vi "Download File to Stream.vi"(6 "timeout (ms)":i32=30000, 8 "error in":errorcluster, 10 "remote path":string, 11 "session in":refnum<class "Session.lvclass">) -> (0 "error out":errorcluster, 2 "channel":T1, 3 "session out":refnum<class "Session.lvclass">)   [LabVIEW 2020, in "NI_SFTP.lvlib"]
doc: "Downloads a remote file, returning the contents as a High-Speed Stream of byte arrays."
uses:
  <vilib>/net/SFTP/NI_SFTP.lvlib
  <vilib>/net/SFTP/Session/Session.lvclass
  <extravilib>/ChannelInstances/High Speed Stream-a[.](u8)/)Channel.ctl
  <vilib>/ChannelSupport/Channel Abort Instructions.ctl
  <extravilib>/ChannelInstances/High Speed Stream-a[.](u8)/)Channel.vi
  <vilib>/net/SFTP/API/Support/Download/Stream/Stream Download Controller.lvclass
  <vilib>/Utility/Deadline/NI_Deadline.lvlib
  <extravilib>/ChannelInstances/High Speed Stream-a[.](u8).lvlib
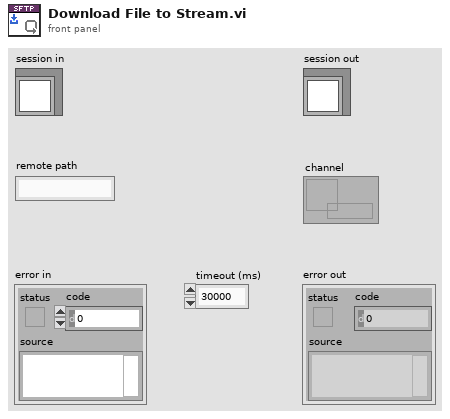
[diagram p1: front panel]
types:
  T1 = typedef "High Speed Stream-a[.](u8).lvlib/)Channel.ctl" = refnum<queue>
  T2 = typedef "Channel Abort Instructions.ctl" = enum16{"No abort", "Abort now", "Abort if timeout"}
  T3 = typedef "NI_Deadline.lvlib/Deadline.ctl" = cluster{"mode":T4, "deadline (ms)":u32}
  T4 = typedef "NI_Deadline.lvlib/Mode.ctl" = enum16{"Relative", "Use deadline", "Wait forever", "Nonblocking", "N/A"}
  T5 = typedef "NI_SFTP.lvlib/Stream Download Controller.lvclass/Element.ctl" = cluster{"data":u8[], "abort":bool}
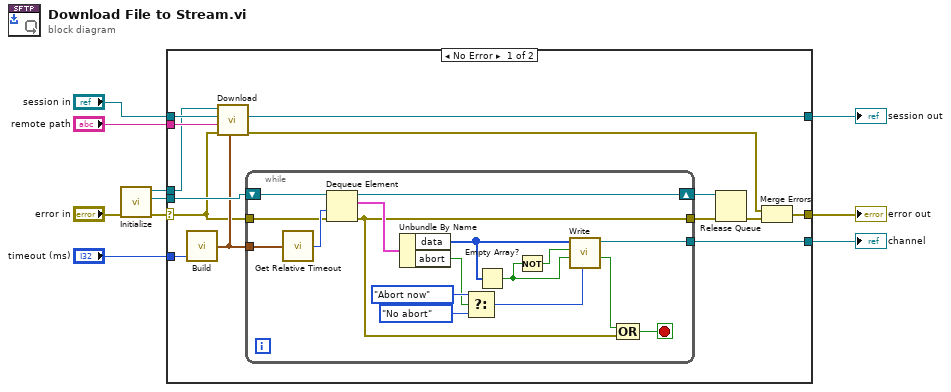
[diagram p0: block diagram]
diagram:
  n1 = call <vilib>:"Initialize.vi"("error in (no error)"="error in") -> ("error out"=w3:errorcluster, "queue out"=w5:refnum<queue>, "Stream Download Controller out"=w6:refnum<class "Stream Download Controller.lvclass">)  [unwired: 8 in]
  n2 = case shown="No Error" w3 {
    selector: w3 -> [w15 w43]
    tunnel: "session in" -> [w24 w42]
    tunnel: "remote path" -> [w23 _]
    tunnel: "timeout (ms)" -> [w22 _]
    tunnel: w6 -> [w21 _]
    tunnel: w5 -> [w20 _]
    tunnel: [w19 _] -> w4
    tunnel: [w12 w42] -> w2
    tunnel: [w11 w43] -> w1
    frame No Error {
      n3 = call <vilib>:"Build.vi"("timeout (ms)"=w22) -> ("Deadline out"=w16:T3)  [unwired: 2 in]
      n4 = call-dynamic "Download.vi"("deadline"=w16, "error in"=w15, "remote path"=w23, "session in"=w24, "NI_SFTP.lvlib:Generic Download Controller.lvclass"=w21) -> ("error out"=w14:errorcluster, "session out"=w12:refnum<class "Session.lvclass">)  [unwired: 4 in, 1 out]
      n5 = while {
        tunnel: [w33] -> w19
        shift-right: [w31] -> w18
        shift-left: w20 -> [w41]
        tunnel: [w28] -> w17
        tunnel: w16 -> [w26]
        tunnel: w15 -> [w25]
        stop <- w29 stop-if-true
        n6 = call <vilib>:"Get Relative Timeout.vi"("Timeout"=w26) -> ("timeout (ms) out"=w27:i32)
        n7 = Dequeue Element(queue=w41, timeout in ms (-1)=w27, error in (no error)=w25) -> (queue out=w31:refnum<queue>, element=w35:T5, error out=w28:errorcluster)  [unwired: 1 out]
        n8 = Unbundle By Name(w35) -> ("data"=w34:u8[], "abort"=w32:bool)
        n9 = Select(t=Channel_Abort_Instructions."Abort now" ("abort status (no abort)"), s=w32, f=Channel_Abort_Instructions."No abort" ("abort status (no abort)")) -> (s? t:f=w36:T2)
        n10 = Empty Array?(array=w34) -> (empty?=w40:bool)
        n11 = Not(x=w40) -> (.not. x?=w39:bool)
        n12 = call <extravilib>:"Write.vi"("abort status (no abort)"=w36, "last element? (F)"=w40, "element valid? (T)"=w39, "element"=w34) -> ("done?"=w30:bool, "channel"=w33:T1)  [unwired: 5 in, 1 out]
        n13 = Compound Arithmetic op=OR(w30, w28) -> (w29:bool)
      }
      n14 = Release Queue(queue=w18, error in (no error)=w17) -> (error out=w13:errorcluster)  [unwired: 1 in, 2 out]
      n15 = Merge Errors(w14, w13) -> (w11:errorcluster)
    }
    frame Error {
    }
  }
  "error out" <- w1
  "session out" <- w2
  "channel" <- w4
